vi "FUG-HCN.SetCurrent.vi"(0 "i ref in":refnum<vi>, 2 "Set Current{mA}":dbl format="%.5f", 3 "Time out":i32, 5 "error in (no error)":errorcluster) -> (14 "i ref out":refnum<vi>, 16 "timed out":bool, 19 "error out":errorcluster)   [LabVIEW 2014, in "FUG-HCN.lvlib"]
doc: "Sets the Current at the device"
uses:
  FUG-HCN.lvlib
  CSCore/CSSystem/CoreDefs/CoreDefs.error_type.ctl
  CSCore/CSSystem/CoreLib/CoreLib.lvlib
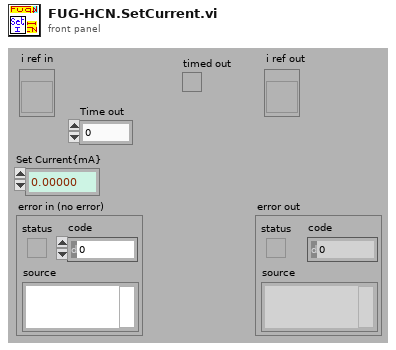
[diagram p1: front panel]
types:
  T1 = cluster{"VISA resource name":refnum<visa-resource-name>, "Gen time out":dbl, "timeout (0)":u32}
  T2 = typedef "CoreDefs.error_type.ctl" = enum16{"no error", "can't load process", "can't unload process", "process does not exist", "can't install process", "can't remove process", "unknown function", "time out", "can't execute function", "duplicate queue name", "super not found", "caller queue invalid", "can't ping process", "unknown error", "VISA Error", "VISA timeout", "GPIB timeout", "GPIB error", "communication error", "data type mismatch", "can't read data from OPC server", "can't write data to OPC server", "OET error", "function not implemented", "process already exists", "invalid Shared Variable name", "error writing Shared Variable", "error reading Shared Variable", "invalid client name", "corrupt database", "unknown class", "call not authorized", "parameter out of range", "OET timeout: can't get data to modify", "invalid queue name", "requested operation incompatible with current state", "event undefined", "event disabled", "state undefined", "caller is not a friend", "EventBuilder: bad eventID", "EventBuilder: no DAQ devices", "a thread must not stop itself", "UNUSED ELEMENT4", "DiscArchiver: eventData incomplete", "DiscArchiver: eventData does not belong to run", "DiscArchiver: can't open file", "DiscArchiver: can't write to file", "DiscArchiver: available disc space low", "can't acquire semaphore", "error reading data from database", "notifier object is not existing", "can't register process", "can't unregister process", "illegal event type", "object disabled", "object already exists", "can't change state", "Instrument not found", "no connection to remote node", "invalid reference", "N/A", "UNUSED ELEMENT 1", "element not found", "illegal TCP/IP connection detected", "object does not exist", "invalid access ID", "unknown CS system", "invalid privilige", "unsupported data type", "unsupported server type", "IO server already exists", "Shared Variable already exists"}
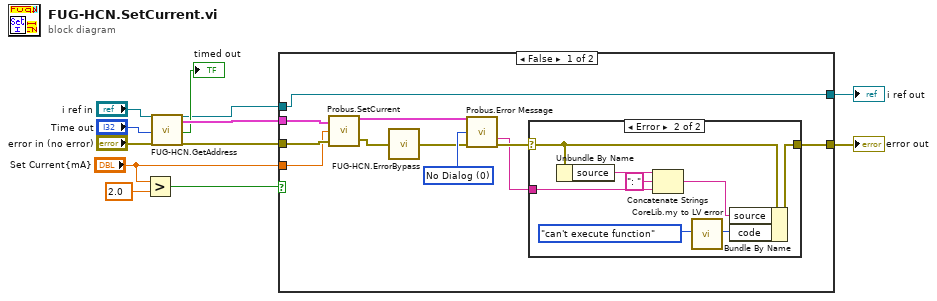
[diagram p0: block diagram]
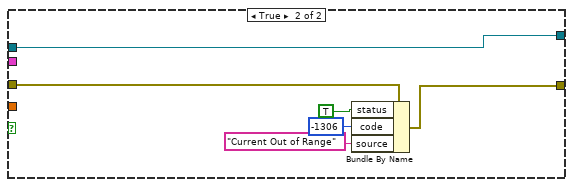
[diagram p3: hidden frame]
diagram:
  n1 = Greater?(x="Set Current{mA}", y=2.0) -> (0:w3:bool)
  n2 = call "FUG-HCN.GetAddress.vi"("i ref in"="i ref in", "Timeout"="Time out", "error in (no error)"="error in (no error)") -> ("i ref out"=w2:refnum<vi>, "VISA cluster out"=w10:T1, "timed out"=→"timed out":bool, "error out"=w9:errorcluster)  [unwired: 13 in]
  n3 = case shown="False" w3 {
    tunnel: w10 -> [w23 _]
    tunnel: w9 -> [w22 w37]
    tunnel: [w21 w36] -> w7
    tunnel: "Set Current{mA}" -> [w16 _]
    tunnel: w2 -> [w15 w38]
    tunnel: [w15 w38] -> w1
    frame False {
      w18 = 0 items=["No Dialog", "OK Message", "Continue or Stop Message"] ("Type of Dialog (1: OK Msg)")
      n4 = call "Probus.SetCurrent.vi"("error in (no error)"=w22, "Set Current{mA}"=w16, "VISA cluster in"=w23) -> ("error out"=w14:errorcluster, "VISA cluster out"=w20:T1)
      n5 = call "FUG-HCN.ErrorBypass.vi"("error in (no error)"=w14) -> ("error out"=w13:errorcluster)  [unwired: 14 in]
      n6 = call "Probus.Error Message.vi"("Visa Cluster in"=w20, "Type of Dialog (1: OK Msg)"=w18, "error in (no error)"=w13) -> ("Error Message (empty)"=w17:string, "error out"=w19:errorcluster)  [unwired: 8 in, 3 out]
      n7 = case shown="Error" w19 {
        selector: w19 -> [w24 w29]
        tunnel: [w24 w31] -> w21
        tunnel: w17 -> [_ w26]
        frame No Error {
        }
        frame Error {
          n8 = Unbundle By Name(w29) -> ("source"=w28:string)
          n9 = Concatenate Strings(w28, ": " ("string"), w26) -> (w25:string)
          n10 = call "CoreLib.my to LV error.vi"("ErrorTypes"=CoreDefs.error_type."can't execute function") -> ("LV error code"=w30:i32)  [unwired: 17 in, 1 out]
          n11 = Bundle By Name(cluster=w29, "source"=w25, "code"=w30) -> (w31:errorcluster)
        }
      }
    }
    frame True {
      n12 = Bundle By Name(cluster=w37, "status"=TRUE, "code"=-1306, "source"="Current Out of Range") -> (w36:errorcluster)
    }
  }
  "error out" <- w7
  "i ref out" <- w1
